vi "paddleOcr_Openvino.vi"() -> ()   [LabVIEW 2018]
uses:
  <vilib>/VIRobotics/opencv_yiku/ctls/Size.ctl
  <vilib>/VIRobotics/opencv_yiku/ctls/ColorConversionCodes.ctl
  <vilib>/VIRobotics/opencv_yiku/ctls/LineTypes.ctl
  <vilib>/VIRobotics/opencv_yiku/Mat/Mat_8U/Mat_8U.lvclass
  C:/Program Files/National Instruments/LabVIEW 2018/vi.lib/VIRobotics/opencv_yiku/Mat/Mat/Mat.lvclass
  <vilib>/VIRobotics/opencv_yiku/geometry/vector_Point/vector_Point_set_points.vi
  <vilib>/VIRobotics/opencv_yiku/geometry/vector_Point/vector_Point_release.vi
  <vilib>/VIRobotics/opencv_yiku/Mat/Mat/Mat_release.vi
  <vilib>/VIRobotics/ModelZoo/PaddleOCR/ppocr_openvino/ppocr_openvino.lvclass
  <vilib>/VIRobotics/opencv_yiku/opencv_yiku.lvlib
  <vilib>/VIRobotics/opencv_yiku/geometry/vector_Point/vector_Point.lvclass
  <vilib>/VIRobotics/opencv_yiku/Mat/Mat/Mat.lvclass
panel:
  in  "stop":bool
  out "time(s)":dbl
  in  "use cls":bool
  in  "backend":string="CPU"
  in  "img_path":path
  in  "model_base_path":path=path "C:/ProgramData/VIRobotics/ModelZoo/PaddleOCR"
  in  "Model Choose":T1(tab)=enum."PPOCRv5_server"
  in  "PPOCRv3-Ch":string[](array[string])=["detect\\det.onnx", "rec\\rec.onnx", "cls\\cls.onnx", "ch_dict.txt"]
  in  "PPOCRv3-En":string[](array[string])=["detect\\det.onnx", "rec\\en_rec.onnx", "cls\\cls.onnx", "en_dict.txt"]
  in  "PPOCRV4":string[](array[string])=["detect\\detv4.onnx", "rec\\recv4.onnx", "cls\\cls.onnx", "ch_dict.txt"]
  in  "PPOCRV5":string[](array[string])=["ppocrv5\\PP-OCRv5_server_det_infer.onnx", "ppocrv5\\PP-OCRv5_server_rec_infer.onnx", "cls\\cls.onnx", "ppocrv5\\ppocrv5_dict.txt"]
  in  "PPOCRV5_mobile":string[](array[string])=["ppocrv5\\PP-OCRv5_mobile_det_infer.onnx", "ppocrv5\\PP-OCRv5_mobile_rec_infer.onnx", "cls\\cls.onnx", "ppocrv5\\ppocrv5_dict.txt"]
  out "result":string[](array[string])
  out "Array":picture[](array[picture])
  in  "scale":dbl=4.0 step=0.1 format="%#_13g"
  out "picture":picture
  # "Running PPOCR with OpenVINO in LabVIEW"
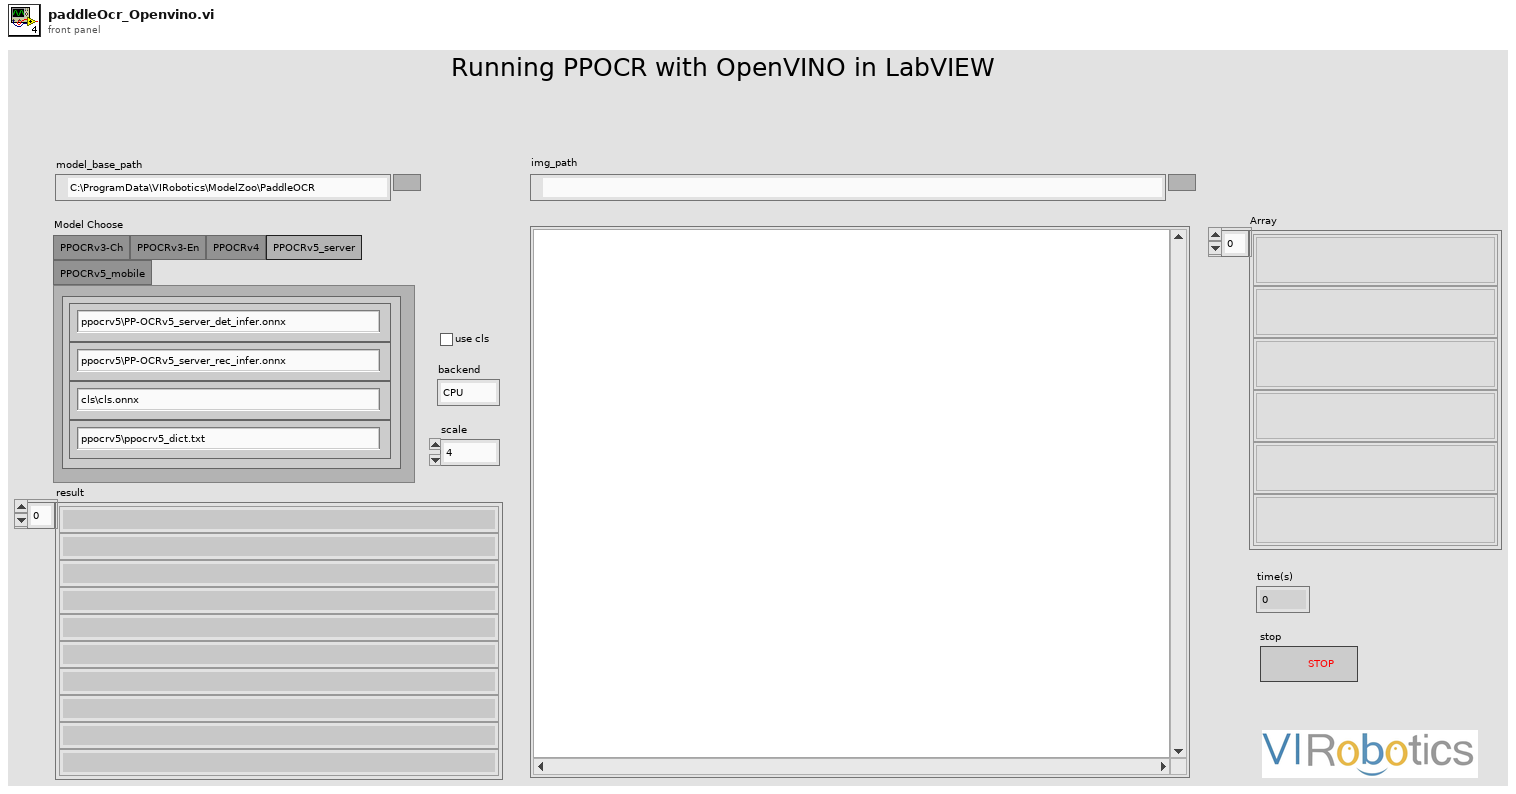
[diagram p1: front panel]
types:
  T1 = enum32{"PPOCRv3-Ch", "PPOCRv3-En", "PPOCRv4", "PPOCRv5_server", "PPOCRv5_mobile"}
  T2 = cluster{"model_path":path, "backend":string, "deviceID":i32}
  T3 = typedef "opencv_yiku.lvlib/Size.ctl" = cluster{"x":i32, "y":i32}
  T4 = cluster{"[0]":cluster{"model_path":path, "backend":string, "deviceID":i32}, "[1]":cluster{"model_path":path, "backend":string, "deviceID":i32}, "[2]":cluster{"model_path":path, "backend":string, "deviceID":i32}, "[3]":cluster{"model_path":path, "backend":string, "deviceID":i32}}
  T5 = typedef "opencv_yiku.lvlib/ColorConversionCodes.ctl" = enum32{"COLOR_BGR2BGRA", "COLOR_BGRA2BGR", "COLOR_BGR2RGBA", "COLOR_RGBA2BGR", "COLOR_BGR2RGB", "COLOR_BGRA2RGBA", "COLOR_BGR2GRAY", "COLOR_RGB2GRAY", "COLOR_GRAY2BGR", "COLOR_GRAY2BGRA", "COLOR_BGRA2GRAY", "COLOR_RGBA2GRAY", "COLOR_BGR2BGR565", "COLOR_RGB2BGR565", "COLOR_BGR5652BGR", "COLOR_BGR5652RGB", "COLOR_BGRA2BGR565", "COLOR_RGBA2BGR565", "COLOR_BGR5652BGRA", "COLOR_BGR5652RGBA", "COLOR_GRAY2BGR565", "COLOR_BGR5652GRAY", "COLOR_BGR2BGR555", "COLOR_RGB2BGR555", "COLOR_BGR5552BGR", "COLOR_BGR5552RGB", "COLOR_BGRA2BGR555", "COLOR_RGBA2BGR555", "COLOR_BGR5552BGRA", "COLOR_BGR5552RGBA", "COLOR_GRAY2BGR555", "COLOR_BGR5552GRAY", "COLOR_BGR2XYZ", "COLOR_RGB2XYZ", "COLOR_XYZ2BGR", "COLOR_XYZ2RGB", "COLOR_BGR2YCrCb", "COLOR_RGB2YCrCb", "COLOR_YCrCb2BGR", "COLOR_YCrCb2RGB", "COLOR_BGR2HSV", "COLOR_RGB2HSV", "42", "43", "COLOR_BGR2Lab", "COLOR_RGB2Lab"}
  T6 = typedef "opencv_yiku.lvlib/LineTypes.ctl" = u16
  T7 = typedef "opencv_yiku.lvlib/Point2f.ctl" = cluster{"x":sgl, "y":sgl}
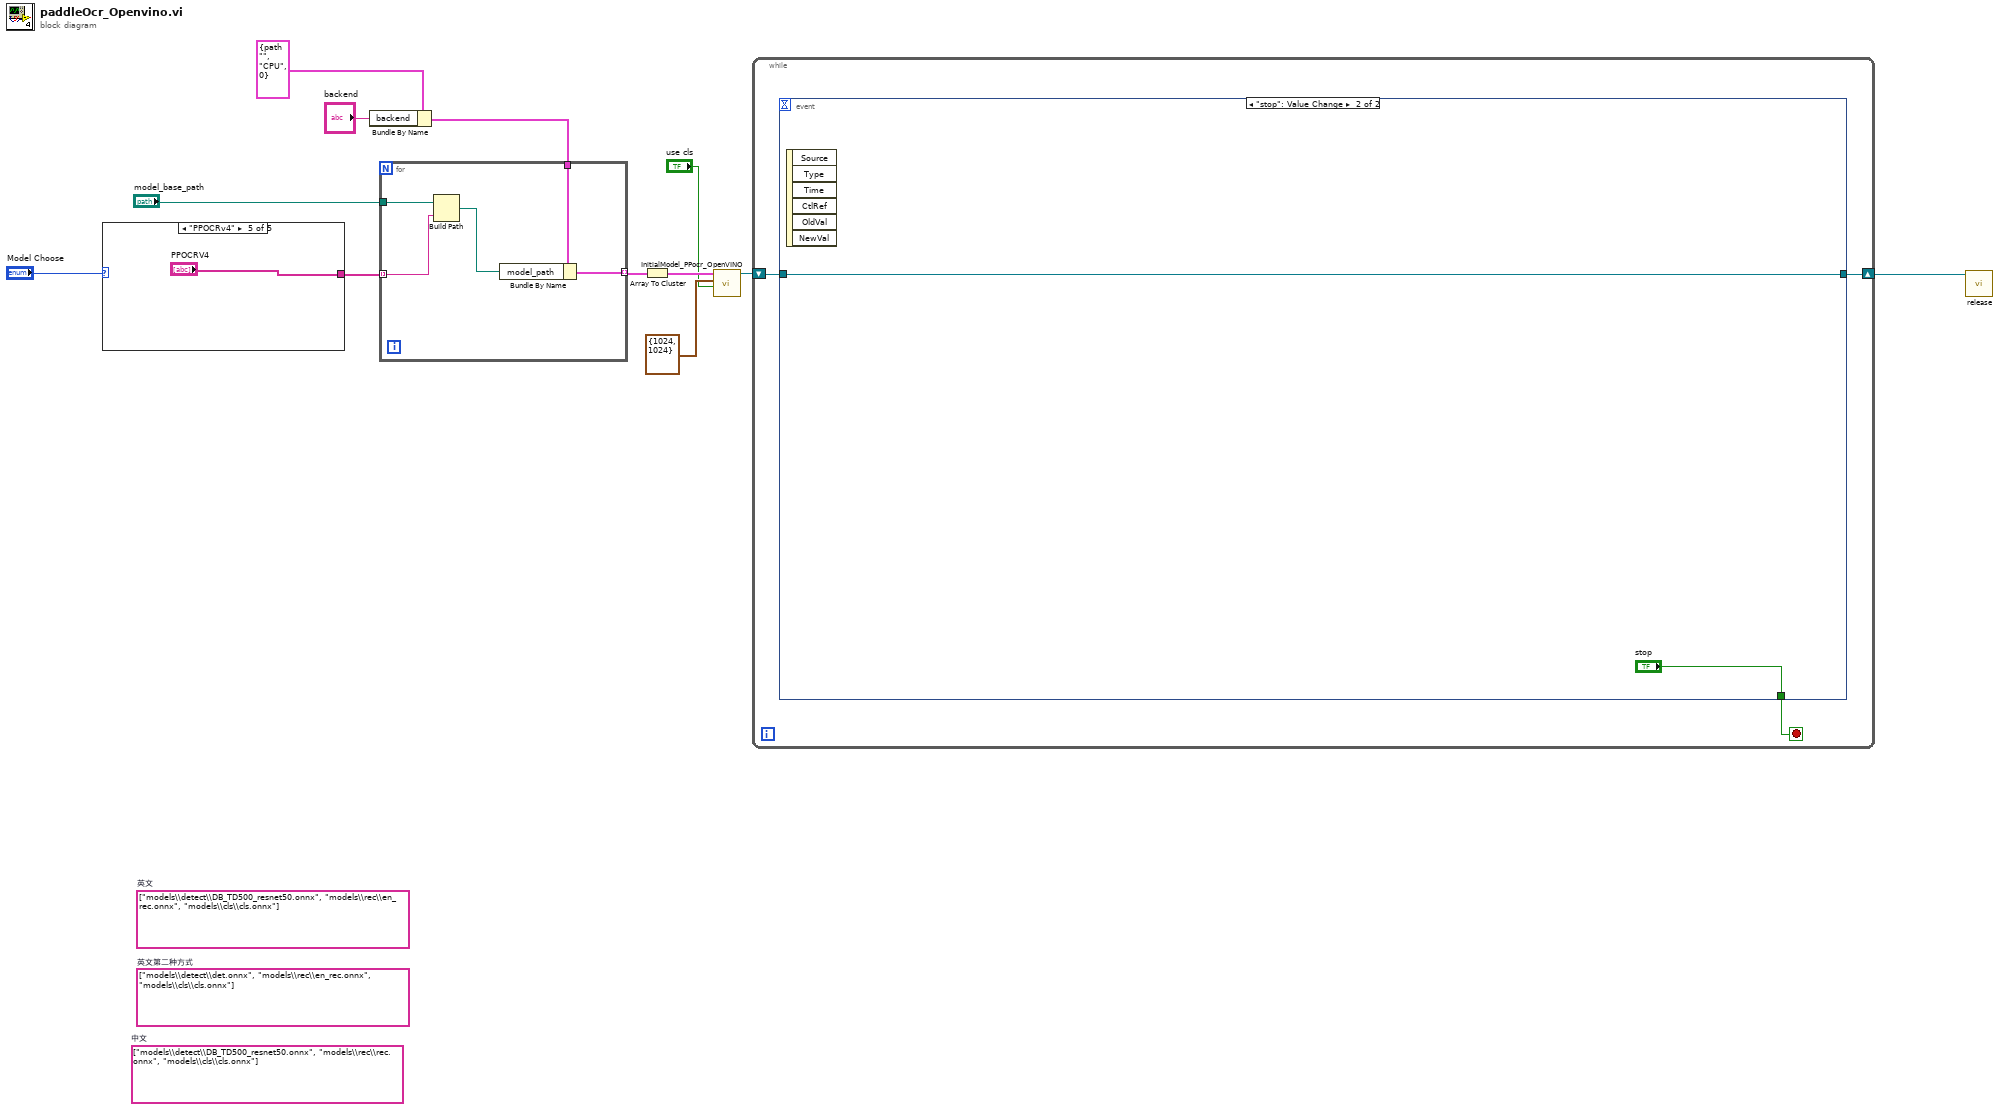
[diagram p0: block diagram]
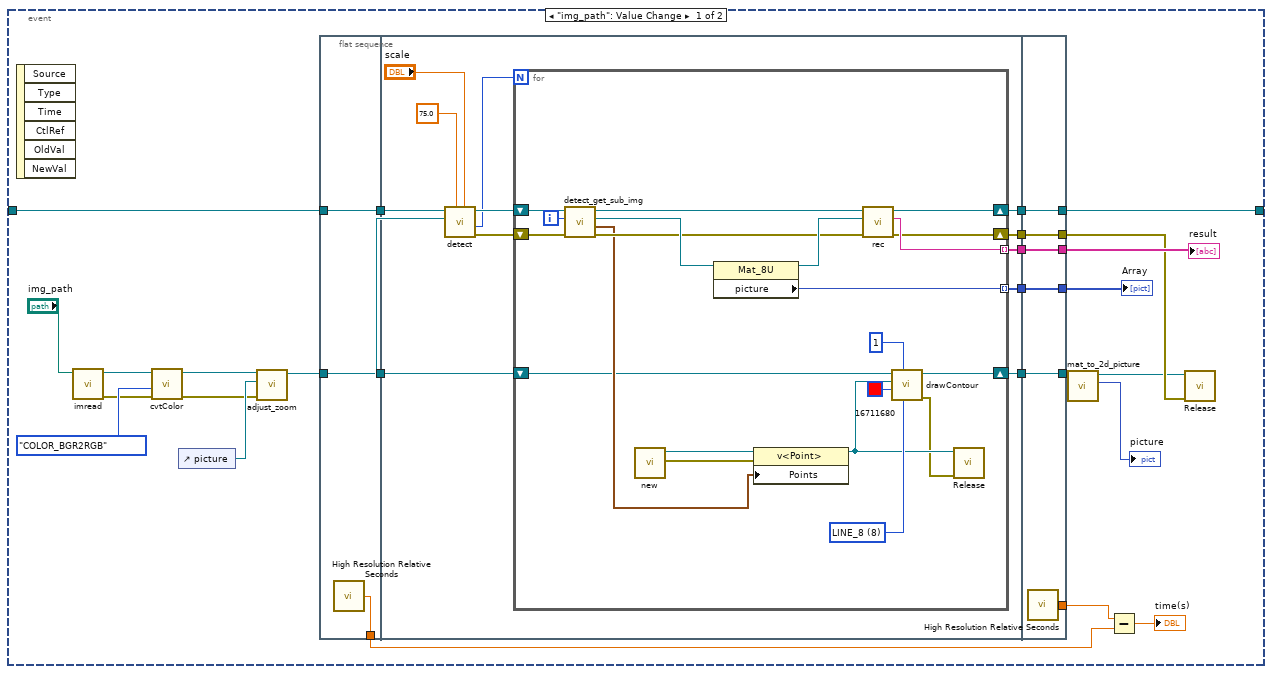
[diagram p2: hidden frame]
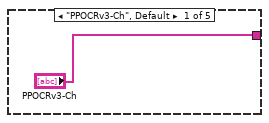
[diagram p3: hidden frame]
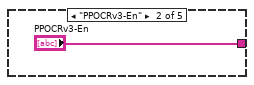
[diagram p4: hidden frame]
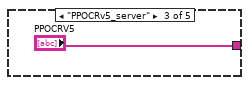
[diagram p5: hidden frame]
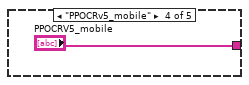
[diagram p6: hidden frame]
diagram:
  (unwired) string[] ["models\\detect\\det.onnx", "models\\rec\\en_rec.onnx", "models\\cls\\cls.onnx"]  # 英文第二种方式
  (unwired) string[] ["models\\detect\\DB_TD500_resnet50.onnx", "models\\rec\\en_rec.onnx", "models\\cls\\cls.onnx"]  # 英文
  (unwired) string[] ["models\\detect\\DB_TD500_resnet50.onnx", "models\\rec\\rec.onnx", "models\\cls\\cls.onnx"]  # 中文
  n1 = case shown="\"PPOCRv4\"" "Model Choose" {
    tunnel: ["PPOCRv3-Ch" "PPOCRv3-En" "PPOCRV5" "PPOCRV5_mobile" "PPOCRV4"] -> w10
    frame "PPOCRv3-Ch", Default {
    }
    frame "PPOCRv3-En" {
    }
    frame "PPOCRv5_server" {
    }
    frame "PPOCRv5_mobile" {
    }
    frame "PPOCRv4" {
    }
  }
  n2 = Bundle By Name(cluster=T2 {"model_path"=path "", "backend"="CPU", "deviceID"=0} ("det"), "backend"="backend") -> (w7:T2)
  n3 = for {
    tunnel: w7 -> [w22]
    tunnel: "model_base_path" -> [w21]
    tunnel: w10 -> [w20] mode=indexing
    tunnel: [w18] -> w12 mode=indexing
    n4 = Build Path(base path=w21, name or relative path=w20) -> (appended path=w19:path)
    n5 = Bundle By Name(cluster=w22, "model_path"=w19) -> (w18:T2)
  }
  n6 = Array To Cluster(array=w12) -> (cluster=w3:T4)
  n7 = call <vilib>:"InitialModel_PPocr_OpenVINO.vi"("use cls"="use cls", "Size"=T3 {"x"=1024, "y"=1024}, "model_info"=w3) -> ("ppocr_onnx out"=w6:refnum<class "ppocr_openvino.lvclass">)  [unwired: 7 in, 1 out]
  n8 = while {
    shift-right: [w24] -> w11
    shift-left: w6 -> [w25]
    stop <- w23 stop-if-true
    n9 = event shown="[1] \"stop\": Value Change" {
      selector: _ -> [_ _]
      dyn-events: _ -> [_ _]
      timeout: _ -> [_ _]
      tunnel: w25 -> [w46 w95]
      tunnel: [w44 w95] -> w24
      tunnel: [_ "stop"] -> w23
      event "img_path": Value Change {
        n10 = event-data() -> ()  [unwired: 1 in, 6 out]
        n11 = call <vilib>:"imread.vi"("path"="img_path") -> ("error out"=w48:errorcluster, "Mat out"=w50:refnum<class "Mat_8U.lvclass">)  [unwired: 9 in]
        n12 = call <vilib>:"cvtColor.vi"("error in (no error)"=w48, "dstCn"=ColorConversionCodes."COLOR_BGR2RGB", "src"=w50) -> ("error out"=w47:errorcluster, "src out"=w45:refnum<class "Mat_8U.lvclass">)  [unwired: 6 in, 1 out]
        n13 = control-ref of="picture"() -> (w51:refnum<vi>)
        n14 = call <vilib>:"adjust_zoom.vi"("error in (no error)"=w47, "picture"=w51, "img"=w45) -> ("img out"=w36:refnum<class "Mat_8U.lvclass">)  [unwired: 7 in, 1 out]
        n15 = flat-sequence {
          tunnel: w36 -> [w53]
          tunnel: w46 -> [w54]
          tunnel: [w54] -> w35
          tunnel: [w53] -> w34
          tunnel: [w52] -> w27
          tunnel: w35 -> [w64]
          tunnel: w34 -> [w55]
          tunnel: [w62] -> w33
          tunnel: [w61] -> w32
          tunnel: [w60] -> w31
          tunnel: [w58] -> w30
          tunnel: [w56] -> w29
          tunnel: [w89] -> w39
          tunnel: [w90] -> w41
          tunnel: [w91] -> w42
          tunnel: [w92] -> w43
          tunnel: [w93] -> w44
          tunnel: w33 -> [w93]
          tunnel: w32 -> [w92]
          tunnel: w31 -> [w91]
          tunnel: w30 -> [w90]
          tunnel: w29 -> [w89]
          tunnel: [w88] -> w28
          frame #0 {
            n16 = call <vilib>:"High Resolution Relative Seconds.vi"() -> ("relative seconds"=w52:dbl)
          }
          frame #1 {
            n17 = call-dynamic "detect.vi"("scale"="scale", "thresh"=75.0, "image"=w55, "OCR_Utils in"=w64) -> ("error out"=w59:errorcluster, "result_size"=w57:i32, "OCR_Utils out"=w63:refnum<class "ppocr_openvino.lvclass">)  [unwired: 4 in, 1 out]
            n18 = for {
              N: w57 -> [_]
              shift-right: [w82] -> w62
              shift-left: w63 -> [w87]
              tunnel: [w84] -> w61 mode=indexing
              tunnel: [w80] -> w60 mode=indexing
              shift-right: [w77] -> w58
              shift-left: w59 -> [w79]
              shift-right: [w69] -> w56
              shift-left: w55 -> [w73]
              i -> [w86]
              w72 = T6 8 items=["FILLED"=0, "LINE_4"=4, "LINE_8"=8, "LINE_16"=16] ("linetype")
              n19 = call-dynamic "detect_get_sub_img.vi"("error in (no error)"=w79, "index"=w86, "OCR_Utils in"=w87) -> ("error out"=w78:errorcluster, "Points"=w74:T7[], "sub_img"=w85:refnum<class "Mat_8U.lvclass">, "OCR_Utils out"=w83:refnum<class "ppocr_openvino.lvclass">)  [unwired: 5 in]
              n20 = call <vilib>:"new.vi"() -> ("error out"=w76:errorcluster, "vector<Point> out"=w75:refnum<class "vector_Point.lvclass">)  [unwired: 10 in]
              n21 = property class="Mat_8U"(reference=w85) -> (reference out=w81:refnum<class "Mat_8U.lvclass">, "picture"=w84:picture)  [unwired: 1 in, 1 out]
              n22 = property class="v<Point>"(reference=w75, error in=w76, "Points"=w74) -> (reference out=w68:refnum<class "vector_Point.lvclass">)  [unwired: 1 out]
              n23 = call-dynamic "rec.vi"("error in (no error)"=w78, "image"=w81, "OCR_Utils in"=w83) -> ("error out"=w77:errorcluster, "text"=w80:string, "OCR_Utils out"=w82:refnum<class "ppocr_openvino.lvclass">)  [unwired: 6 in]
              n24 = call <vilib>:"drawContour.vi"("linetype"=w72, "thickness"=1, "Color"=u32 16711680, "vector<Point> in"=w68, "Mat in"=w73) -> ("error out"=w67:errorcluster, "Mat out"=w69:refnum<class "Mat_8U.lvclass">)  [unwired: 5 in]
              n25 = call-poly <vilib>:"Release.vi"("error in (no error)"=w67, "vector<Point> in"=w68) -> ()  [unwired: 9 in, 1 out]
            }
          }
          frame #2 {
            n26 = call <vilib>:"High Resolution Relative Seconds.vi"() -> ("relative seconds"=w88:dbl)
          }
        }
        n27 = call <vilib>:"mat_to_2d_picture.vi"("Mat_8U in"=w39) -> ("picture"=→"picture":picture, "Mat_8U out"=w37:refnum<class "Mat_8U.lvclass">)  [unwired: 8 in, 1 out]
        n28 = Subtract(x=w28, y=w27) -> (x-y=→"time(s)":dbl)
        n29 = call-poly <vilib>:"Release.vi"("error in (no error)"=w41, "Mat in"=w37) -> ()  [unwired: 9 in, 1 out]
        "Array" <- w43
        "result" <- w42
      }
      event "stop": Value Change {
        n30 = event-data() -> ()  [unwired: 1 in, 6 out]
      }
    }
  }
  n31 = call-dynamic <vilib>:"release.vi"("OCR_Utils in"=w11) -> ()  [unwired: 9 in, 2 out]
